vi "Main.vi"(8 "error in":errorcluster) -> (0 "error out":errorcluster)   [LabVIEW 2018, in "Covers-o-meter.lvlib"]
doc: "This module is a free standing module of the car wash.\nIt can be stopped by the 'stop all' user event and has \na QMH architcture. The controller communicates with\nit via its named queue."
uses:
  Covers-o-meter.lvlib
  Private/ctl/Start pause toggle button--boolean.ctl
  Private/ctl/State--enum.ctl
  Private/ctl/Project--cluster.ctl
  Private/ctl/Requirements--cluster.ctl
  <vilib>/National Instruments/Simple DVR Timer API/Timer.lvclass
  Private/ctl/Queue action--enum.ctl
  <vilib>/NI/Timer/Timer Session.lvclass
panel:
  in  "Scan period (min)":dbl[unit]=300.0 format="%#_13g"
  out "Tree 2":string[](tree)
  in  "Reset Button":bool
  out "Cluster":T3
  out "Time left":string
  out "State":T4
  in  "Projects":u16(ring) items=["Car_wash_attempt_2_LE.lvproj", "CLA Covers-o-meter.lvproj"]
  in  "In progress?":T5
  in  "Path to Requirements Tags":path=path "C:/Users/theta/OneDrive/Desktop/CLA/Tools/Sandbox/Data/ATM Requirements Tag.txt"
  out "Coverage over time":waveform(dbl)(graph)
  out "Requirements covered":i32(knob) scale=0.0..103.0
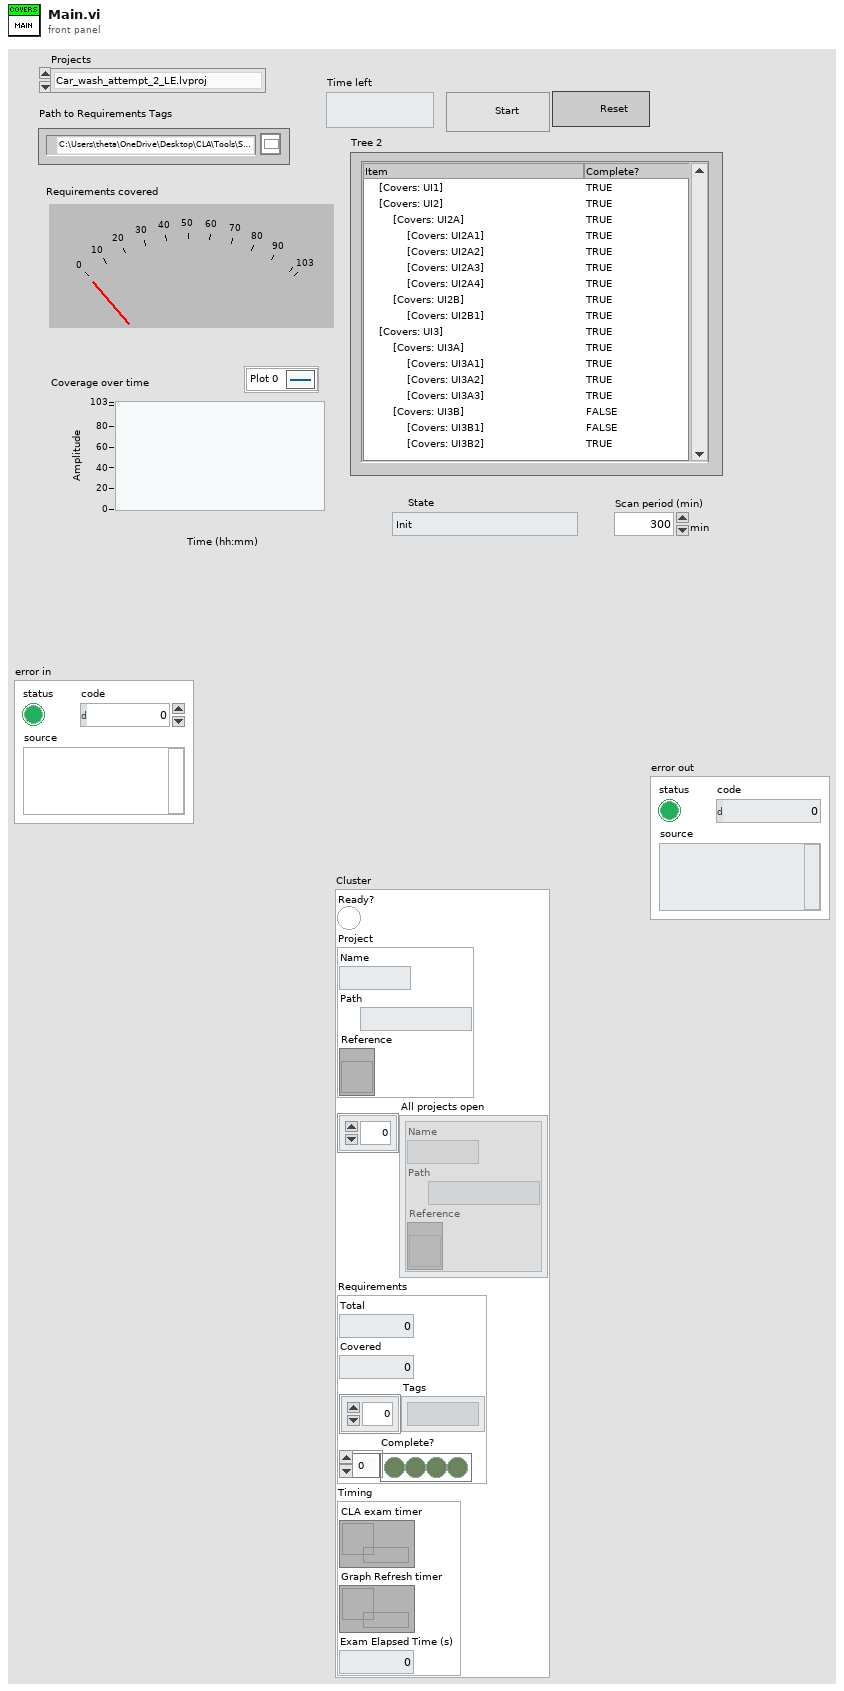
[diagram p1: front panel]
types:
  T1 = typedef "Covers-o-meter.lvlib/Project--cluster.ctl" = cluster{"Name":string, "Path":path, "Reference":refnum<vi>}
  T2 = typedef "Covers-o-meter.lvlib/Requirements--cluster.ctl" = cluster{"Total":i32, "Covered":i32, "Tags":string[], "Complete?":bool[]}
  T3 = cluster{"Ready?":bool, "Project":T1, "All projects open":T1[], "Requirements":T2, "Timing":cluster{"CLA exam timer":refnum<data-value>, "Graph Refresh timer":refnum<data-value>, "Exam Elapsed Time (s)":dbl}}
  T4 = typedef "Covers-o-meter.lvlib/State--enum.ctl" = enum16{"Init", "Init: Read req tags", "Init Data: All Projects", "Init: Which Project?", "Update Requirements tags", "Get all project strings", "Search proj for tags", "Subroutine", "Update Project", "Start Button Pressed", "Start timer", "Error", "Close", "UI - Refresh Timer ", "UI - refresh graph", "UI - Refresh Tree"}
  T5 = typedef "Covers-o-meter.lvlib/Start pause toggle button--boolean.ctl" = bool
  T6 = cluster{"VI Description":bool, "Project Description":bool, "Library Description":bool, "Text within VI":bool, "Class Description":bool}
  T7 = typedef "Covers-o-meter.lvlib/Queue action--enum.ctl" = enum16{"Create", "Get", "Destroy"}
  T8 = typedef "Covers-o-meter.lvlib/Message--enum.ctl" = cluster{"State":T4, "Data":variant}
  T9 = enum8{"Enabled", "Disabled", "Disabled and Grayed Out"}
  T10 = typedef "Start pause toggle button--boolean.ctl" = bool
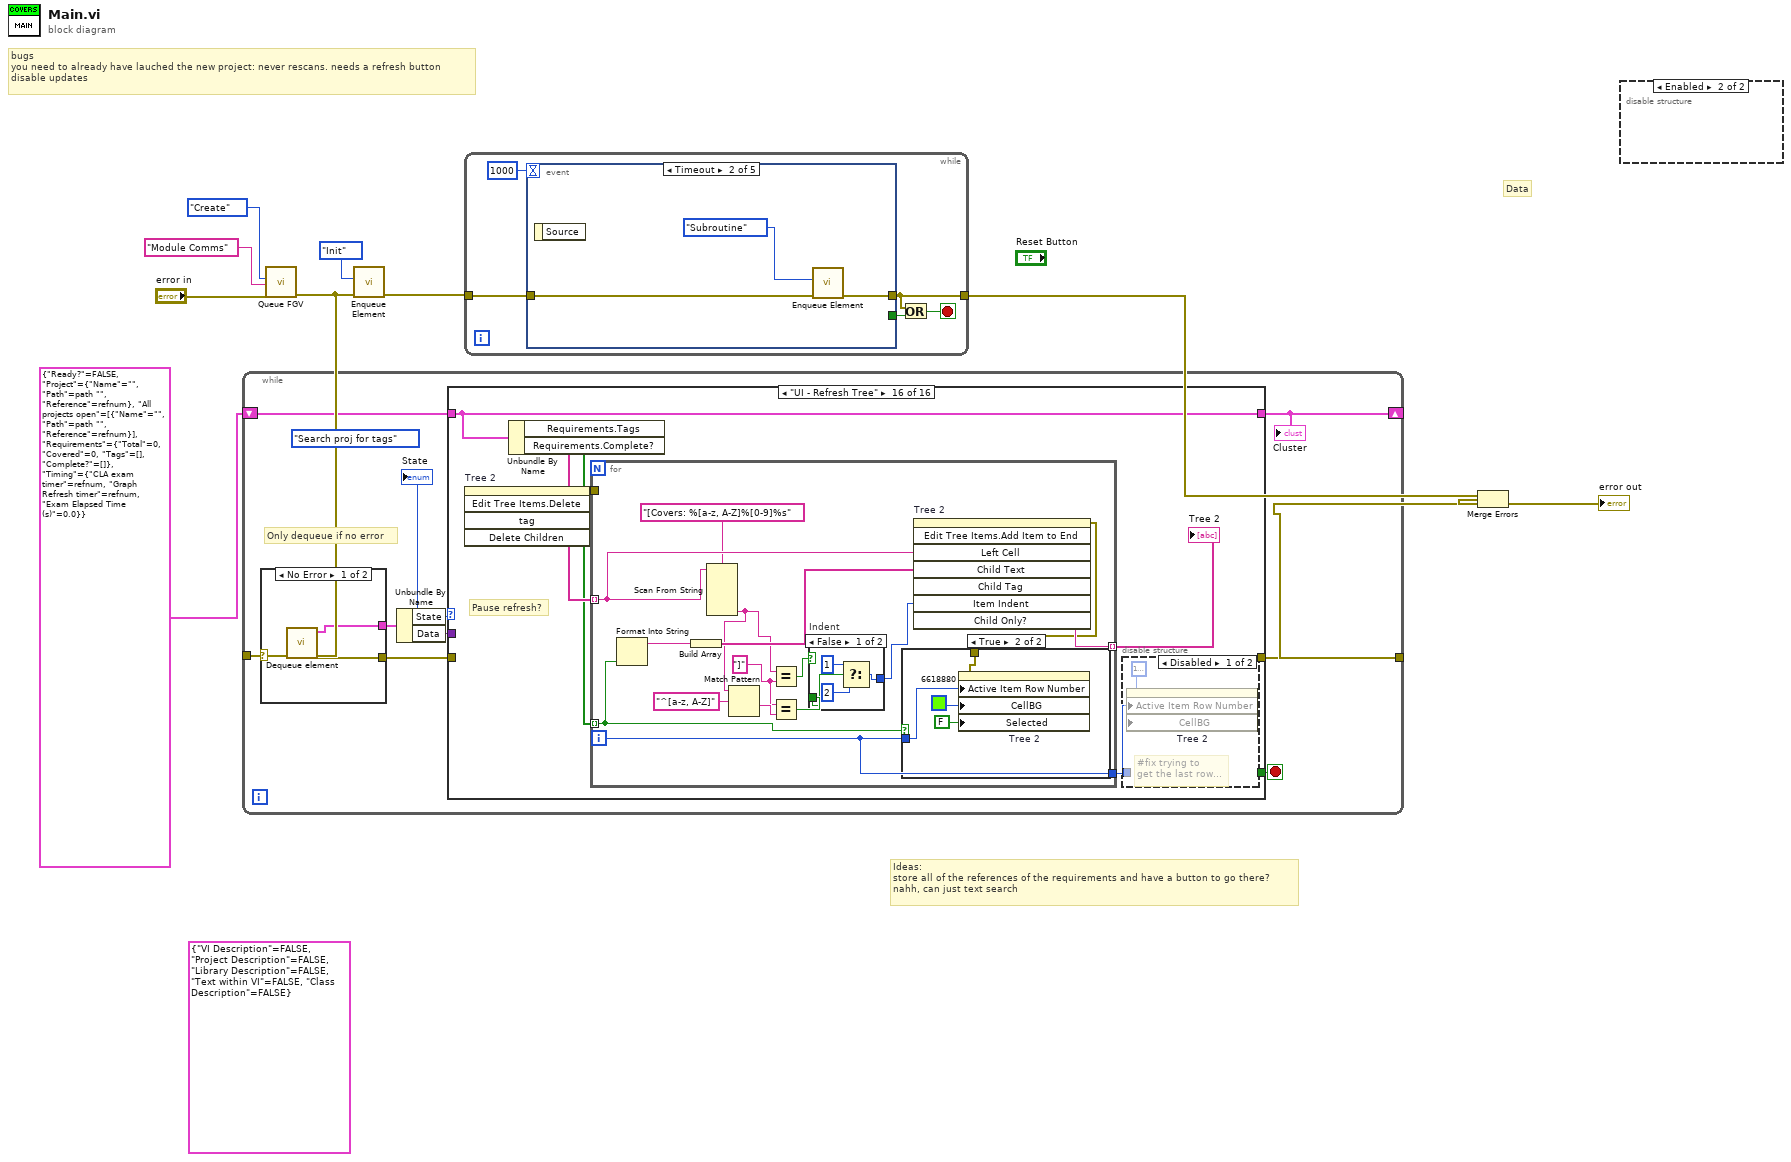
[diagram p0: block diagram]
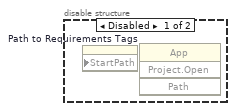
[diagram p2: hidden frame]
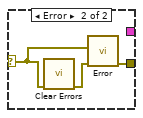
[diagram p3: hidden frame]
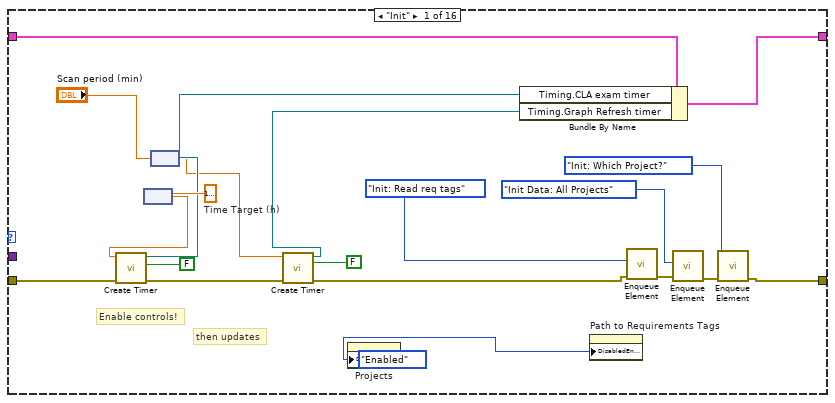
[diagram p4: hidden frame]
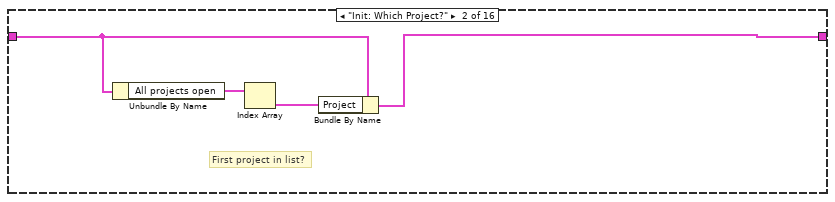
[diagram p5: hidden frame]
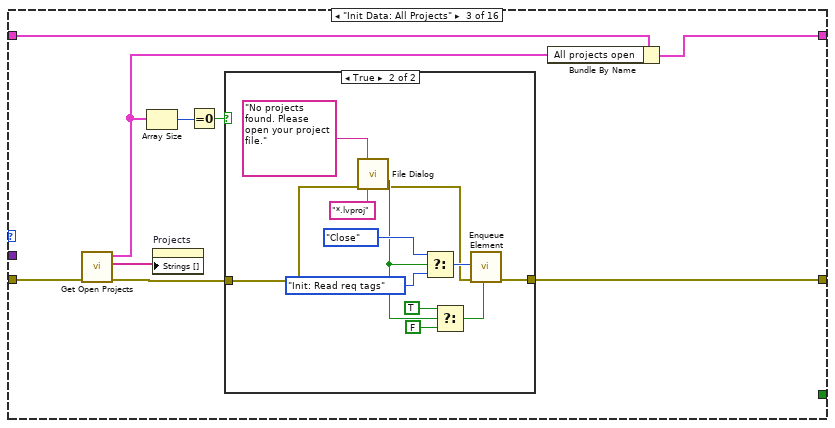
[diagram p6: hidden frame]
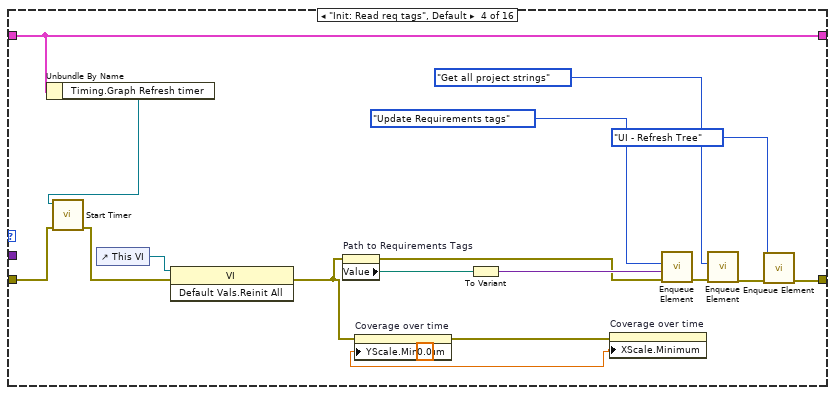
[diagram p8: hidden frame]
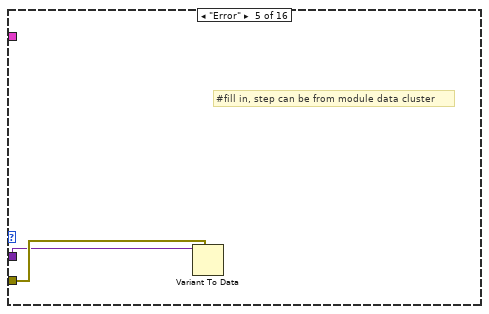
[diagram p9: hidden frame]
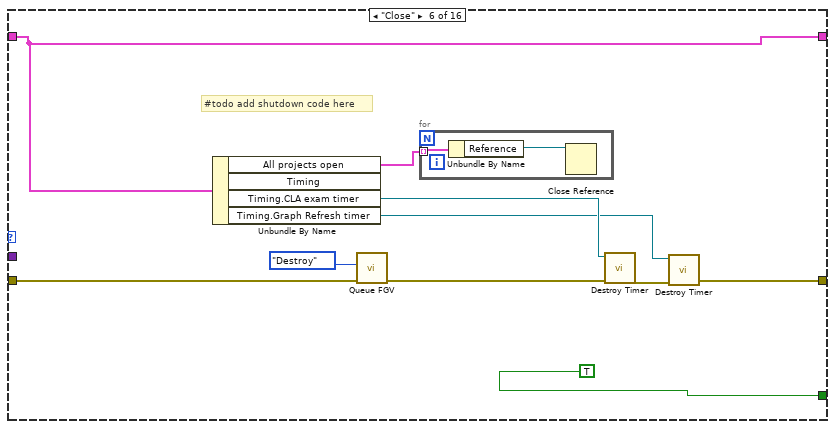
[diagram p10: hidden frame]
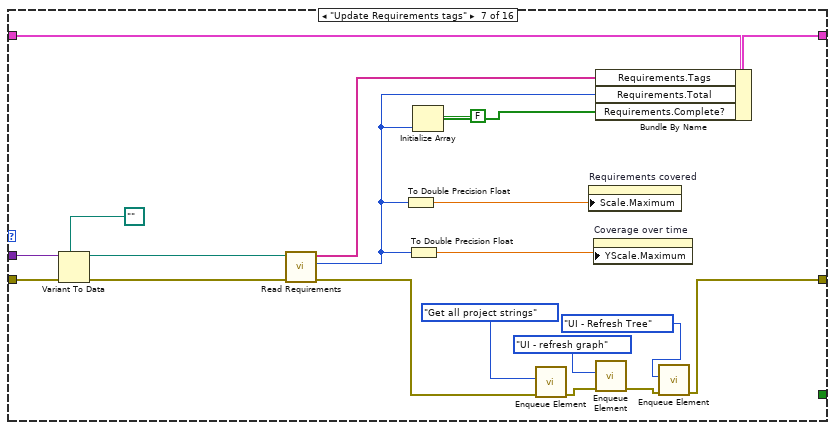
[diagram p11: hidden frame]
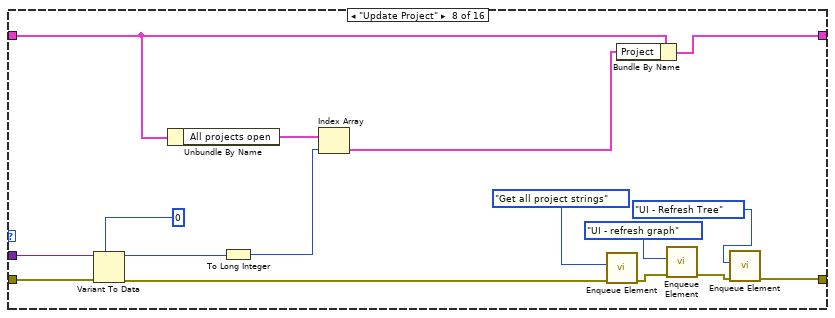
[diagram p12: hidden frame]
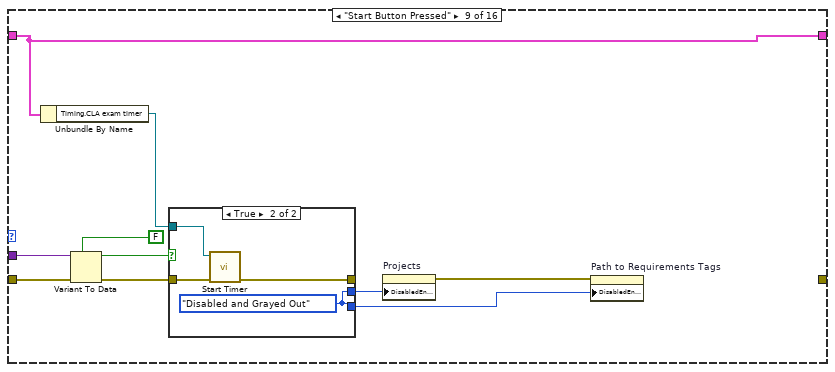
[diagram p13: hidden frame]
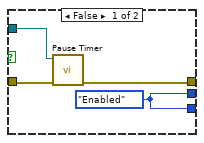
[diagram p14: hidden frame]
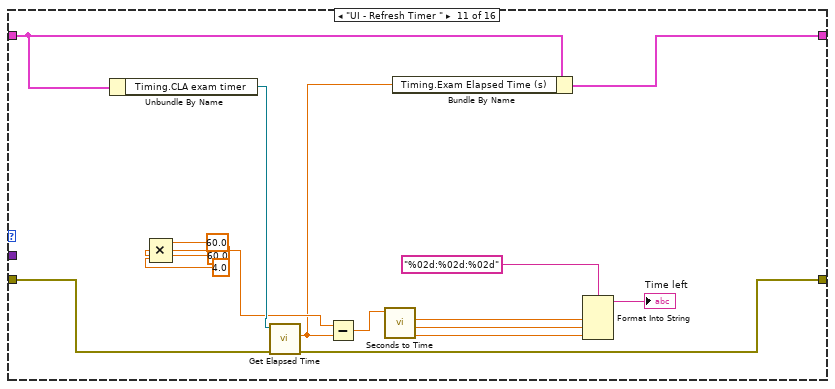
[diagram p16: hidden frame]
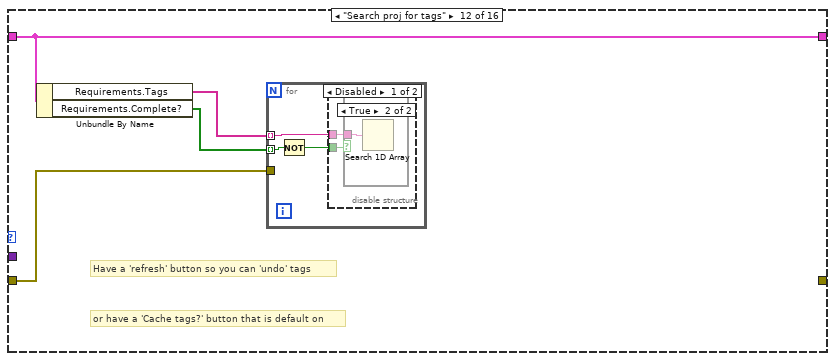
[diagram p17: hidden frame]
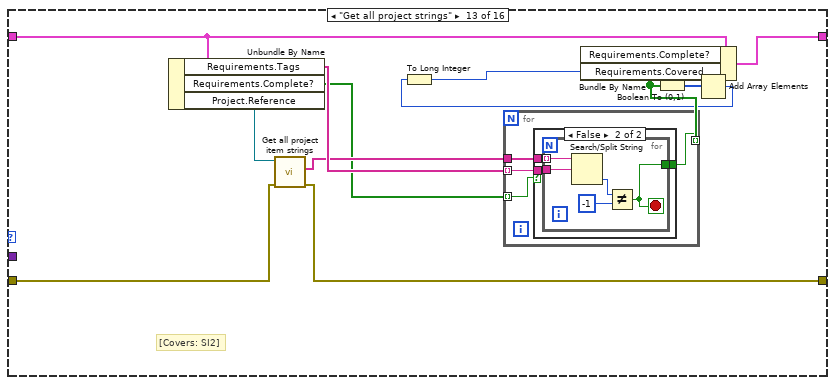
[diagram p20: hidden frame]
diagram:
  (unwired) T6 {"VI Description"=FALSE, "Project Description"=FALSE, "Library Description"=FALSE, "Text within VI"=FALSE, "Class Description"=FALSE}
  # "bugs\nyou need to already have lauched the new project: never rescans. needs a refresh button\ndisable updates"
  # "Ideas:\nstore all of the references of the requirements and have a button to go there?\nnahh, can just text search"
  # "Data"
  n1 = call "Queue FGV.vi"("error in"="error in", "Queue name (unnamed)"="Module Comms", "Queue Action"=Queue_action--enum."Create") -> ("error out"=w7:errorcluster)  [unwired: 7 in, 1 out]
  n2 = while {
    tunnel: [w16] -> w1
    shift-right: [w11] -> _
    shift-left: T3 {"Ready?"=FALSE, "Project"={"Name"="", "Path"=path "", "Reference"=refnum}, "All projects open"=[{"Name"="", "Path"=path "", "Reference"=refnum}], "Requirements"={"Total"=0, "Covered"=0, "Tags"=[], "Complete?"=[]}, "Timing"={"CLA exam timer"=refnum, "Graph Refresh timer"=refnum, "Exam Elapsed Time (s)"=0.0}} -> [w12]
    tunnel: w7 -> [w13]
    stop <- w15 stop-if-true
    (unwired) State--enum."Search proj for tags" ("State")
    # "Only dequeue if no error"
    n3 = case shown="No Error" w13 {
      selector: w13 -> [w21 w23]
      tunnel: [w22 w25] -> w17
      tunnel: [w20 _] -> w19
      frame No Error {
        n4 = call "Dequeue element.vi"("error in (no error)"=w21) -> ("error out"=w22:errorcluster, "Message"=w20:T8)  [unwired: 9 in]
      }
      frame Error {
        n5 = call <vilib>:"Clear Errors.vi"("error in (no error)"=w23) -> ("error out"=w24:errorcluster)  [unwired: 5 in, 1 out]
        n6 = call "Error.vi"("error in (no error)"=w24, "error to pass"=w23) -> ("error out"=w25:errorcluster)  [unwired: 9 in]
      }
    }
    n7 = Unbundle By Name(w19) -> ("State"=w18:T4, "Data"=w14:variant)
    "State" <- w18
    n8 = case shown="\"UI - Refresh Tree\"" w18 {
      tunnel: w17 -> [w40 _ w56 w78 w90 w99 w120 w138 w147 _ w162 w176 w184 w212 w238 _]
      tunnel: [w41 _ w51 w74 _ w91 w103 w124 _ _ w161 _ w195 w213 w237 _] -> w16
      tunnel: [_ _ _ _ _ TRUE _ _ _ _ _ _ _ _ _ _] -> w15
      tunnel: w14 -> [_ _ _ _ w89 _ w121 w137 w146 _ _ _ _ _ _ _]
      tunnel: [w35 w46 w50 w81 _ w95 w117 w132 w142 w157 w158 w174 w190 w217 w235 w242] -> w11
      tunnel: w12 -> [w34 w49 w57 w81 _ w95 w116 w134 w142 w157 w159 w174 w194 w217 w235 w242]
      frame "Init" {
        w26 = T9."Enabled" ("Disabled")
        w39 = dbl[unit] 14400.0  # Time Target (h)
        # "Enable controls!"
        # "then updates"
        n9 = node(w39) -> (w38:dbl)
        n10 = call <vilib>:"Create Timer.vi"("Error In"=w40, "Auto-reset on Time Elapsed"=FALSE, "Time Goal (s)"=w38) -> ("Error Out"=w29:errorcluster, "Timer Reference"=w36:refnum<data-value>)  [unwired: 7 in]
        n11 = node("Scan period (min)") -> (w30:dbl)
        n12 = call <vilib>:"Create Timer.vi"("Error In"=w29, "Auto-reset on Time Elapsed"=FALSE, "Time Goal (s)"=w30) -> ("Error Out"=w32:errorcluster, "Timer Reference"=w27:refnum<data-value>)  [unwired: 7 in]
        n13 = property on="Projects" class="Ring (strict)"("DisabledEnum"=w26) -> ()  [unwired: 2 in, 2 out]
        n14 = Bundle By Name(cluster=w34, "Timing.CLA exam timer"=w36, "Timing.Graph Refresh timer"=w27) -> (w35:T3)
        n15 = property on="Path to Requirements Tags" class="Path"("DisabledEnum"=w26) -> ()  [unwired: 2 in, 2 out]
        n16 = call "Enqueue Element.vi"("error in"=w32, "State"=State--enum."Init: Read req tags") -> ("error out"=w33:errorcluster)  [unwired: 9 in]
        n17 = call "Enqueue Element.vi"("error in"=w33, "State"=State--enum."Init Data: All Projects") -> ("error out"=w43:errorcluster)  [unwired: 9 in]
        n18 = call "Enqueue Element.vi"("error in"=w43, "State"=State--enum."Init: Which Project?") -> ("error out"=w41:errorcluster)  [unwired: 9 in]
      }
      frame "Init: Which Project?" {
        # "First project in list?"
        n19 = Unbundle By Name(w49) -> ("All projects open"=w48:T1[])
        n20 = Index Array(array=w48) -> (element=w47:T1)  [unwired: 1 in]
        n21 = Bundle By Name(cluster=w49, "Project"=w47) -> (w46:T3)
      }
      frame "Init Data: All Projects" {
        n22 = call "Get Open Projects.vi"("error in (no error)"=w56) -> ("error out"=w52:errorcluster, "Project Names"=w58:string[], "Project Data"=w55:T1[])  [unwired: 8 in]
        n23 = Array Size(array=w55) -> (size(s)=w54:i32)
        n24 = property on="Projects" class="Ring (strict)"("Strings []"=w58) -> ()  [unwired: 2 in, 2 out]
        n25 = Equal To 0?(x=w54) -> (x = 0?=w53:bool)
        n26 = case shown="True" w53 {
          tunnel: w52 -> [w59 w62]
          tunnel: [w59 w60] -> w51
          frame False {
            # "It's okay, there's\na project open"
          }
          frame True {
            n27 = call "File Dialog"("prompt"="No projects found. Please open your project file.", "error in"=w62, "pattern (all files)"="*.lvproj") -> ("cancelled"=w66:bool, "error out"=w61:errorcluster)  [unwired: 9 in, 2 out]
            n28 = Select(t=State--enum."Close" ("State"), s=w66, f=State--enum."Init: Read req tags" ("State")) -> (s? t:f=w67:T4)
            n29 = Select(t=TRUE, s=w66, f=FALSE) -> (s? t:f=w64:bool)
            n30 = call "Enqueue Element.vi"("Priority? (F)"=w64, "error in"=w61, "State"=w67) -> ("error out"=w60:errorcluster)  [unwired: 8 in]
          }
        }
        n31 = Bundle By Name(cluster=w57, "All projects open"=w55) -> (w50:T3)
      }
      frame "Init: Read req tags", Default {
        w76 = 0.0 ("Y Scale.Range:Minimum")
        n32 = Unbundle By Name(w81) -> ("Timing.Graph Refresh timer"=w80:refnum<data-value>)
        n33 = call <vilib>:"Start Timer.vi"("Error In"=w78, "Timer Reference"=w80) -> ("Error Out"=w79:errorcluster)  [unwired: 8 in, 1 out]
        n34 = control-ref of="This VI"() -> (w88:refnum<vi>)
        n35 = invoke class="VI" method="Default Vals.Reinit All"(reference=w88, error in=w79) -> (error out=w77:errorcluster)  [unwired: 1 in, 2 out]
        n36 = property on="Path to Requirements Tags" class="Path"(error in=w77) -> (error out=w84:errorcluster, "Value"=w85:path)  [unwired: 1 in, 1 out]
        n37 = property on="Coverage over time" class="WFChart (strict)"(error in=w77, "YScale.Minimum"=w76) -> (error out=w75:errorcluster)  [unwired: 1 in, 1 out]
        n38 = To Variant(anything=w85) -> (Variant=w87:variant)
        n39 = property on="Coverage over time" class="WFChart (strict)"(error in=w75, "XScale.Minimum"=w76) -> ()  [unwired: 1 in, 2 out]
        n40 = call "Enqueue Element.vi"("error in"=w84, "Data"=w87, "State"=State--enum."Update Requirements tags") -> ("error out"=w83:errorcluster)  [unwired: 8 in]
        n41 = call "Enqueue Element.vi"("error in"=w83, "State"=State--enum."Get all project strings") -> ("error out"=w73:errorcluster)  [unwired: 9 in]
        n42 = call "Enqueue Element.vi"("error in"=w73, "State"=State--enum."UI - Refresh Tree") -> ("error out"=w74:errorcluster)  [unwired: 9 in]
      }
      frame "Error" {
        # "#fill in, step can be from module data cluster"
        n43 = Variant To Data(type=w90, Variant=w89) -> ()  [unwired: 1 in, 2 out]
      }
      frame "Close" {
        # "#todo add shutdown code here"
        n44 = Unbundle By Name(w95) -> ("All projects open"=w92:T1[], "Timing.CLA exam timer"=w97:refnum<data-value>, "Timing.Graph Refresh timer"=w93:refnum<data-value>)  [unwired: 1 out]
        n45 = call "Queue FGV.vi"("error in"=w99, "Queue Action"=Queue_action--enum."Destroy") -> ("error out"=w96:errorcluster)  [unwired: 8 in, 1 out]
        n46 = for {
          tunnel: w92 -> [w102] mode=indexing
          n47 = Unbundle By Name(w102) -> ("Reference"=w101:refnum<vi>)
          n48 = Close Reference(reference=w101) -> ()  [unwired: 1 in, 1 out]
        }
        n49 = call <vilib>:"Destroy Timer.vi"("Error In"=w96, "Timer In"=w97) -> ("Error Out"=w94:errorcluster)  [unwired: 8 in, 1 out]
        n50 = call <vilib>:"Destroy Timer.vi"("Error In"=w94, "Timer In"=w93) -> ("Error Out"=w91:errorcluster)  [unwired: 8 in, 1 out]
      }
      frame "Update Requirements tags" {
        n51 = Variant To Data(error in=w120, type=path "", Variant=w121) -> (data=w119:path, error out=w118:errorcluster)
        n52 = call "Read Requirements.vi"("error in (no error)"=w118, "Requirements file"=w119) -> ("error out"=w104:errorcluster, "# Requirements"=w110:i32, "Requirements"=w115:string[])  [unwired: 7 in]
        n53 = To Double Precision Float(number=w110) -> (double precision float=w112:dbl)
        n54 = To Double Precision Float(number=w110) -> (double precision float=w111:dbl)
        n55 = Initialize Array(FALSE, w110) -> (w114:bool[])
        n56 = call "Enqueue Element.vi"("error in"=w104, "State"=State--enum."Get all project strings") -> ("error out"=w106:errorcluster)  [unwired: 9 in]
        n57 = property on="Requirements covered" class="Knob (strict)"("Scale.Maximum"=w112) -> ()  [unwired: 2 in, 2 out]
        n58 = property on="Coverage over time" class="WFChart (strict)"("YScale.Maximum"=w111) -> ()  [unwired: 2 in, 2 out]
        n59 = Bundle By Name(cluster=w116, "Requirements.Tags"=w115, "Requirements.Total"=w110, "Requirements.Complete?"=w114) -> (w117:T3)
        n60 = call "Enqueue Element.vi"("error in"=w106, "State"=State--enum."UI - refresh graph") -> ("error out"=w108:errorcluster)  [unwired: 9 in]
        n61 = call "Enqueue Element.vi"("error in"=w108, "State"=State--enum."UI - Refresh Tree") -> ("error out"=w103:errorcluster)  [unwired: 9 in]
      }
      frame "Update Project" {
        n62 = Variant To Data(error in=w138, type=u16 0 ("NewVal"), Variant=w137) -> (data=w130:u16, error out=w125:errorcluster)
        n63 = Unbundle By Name(w134) -> ("All projects open"=w135:T1[])
        n64 = To Long Integer(number=w130) -> (32bit integer=w131:i32)
        n65 = Index Array(array=w135, index=w131) -> (element=w133:T1)
        n66 = call "Enqueue Element.vi"("error in"=w125, "State"=State--enum."Get all project strings") -> ("error out"=w126:errorcluster)  [unwired: 9 in]
        n67 = Bundle By Name(cluster=w134, "Project"=w133) -> (w132:T3)
        n68 = call "Enqueue Element.vi"("error in"=w126, "State"=State--enum."UI - refresh graph") -> ("error out"=w128:errorcluster)  [unwired: 9 in]
        n69 = call "Enqueue Element.vi"("error in"=w128, "State"=State--enum."UI - Refresh Tree") -> ("error out"=w124:errorcluster)  [unwired: 9 in]
      }
      frame "Start Button Pressed" {
        n70 = Unbundle By Name(w142) -> ("Timing.CLA exam timer"=w143:refnum<data-value>)
        n71 = Variant To Data(error in=w147, type=FALSE, Variant=w146) -> (data=w144:bool, error out=w148:errorcluster)
        n72 = case shown="True" w144 {
          tunnel: [w152 w156] -> _
          tunnel: w148 -> [w151 w155]
          tunnel: w143 -> [w150 w154]
          tunnel: [w149 w153] -> w140
          tunnel: [w149 w153] -> w139
          frame False {
            w149 = T9."Enabled" ("Disabled")
            n73 = call <vilib>:"Pause Timer.vi"("Error In"=w151, "Timer Reference"=w150) -> ("Error Out"=w152:errorcluster)  [unwired: 8 in, 1 out]
          }
          frame True {
            w153 = T9."Disabled and Grayed Out" ("Disabled")
            n74 = call <vilib>:"Start Timer.vi"("Error In"=w155, "Timer Reference"=w154) -> ("Error Out"=w156:errorcluster)  [unwired: 8 in, 1 out]
          }
        }
        n75 = property on="Projects" class="Ring (strict)"("DisabledEnum"=w140) -> (error out=w141:errorcluster)  [unwired: 2 in, 1 out]
        n76 = property on="Path to Requirements Tags" class="Path"(error in=w141, "DisabledEnum"=w139) -> ()  [unwired: 1 in, 2 out]
      }
      frame "Start timer" {
      }
      frame "UI - Refresh Timer " {
        n77 = Unbundle By Name(w159) -> ("Timing.CLA exam timer"=w172:refnum<data-value>)
        n78 = Compound Arithmetic op=MULTIPLY(60.0 ("value"), 60.0 ("value"), 4.0 ("value")) -> (w163:dbl)
        n79 = call <vilib>:"Get Elapsed Time.vi"("Error In"=w162, "Timer Reference"=w172) -> ("Error Out"=w161:errorcluster, "Elapsed Time (s)"=w160:dbl)  [unwired: 6 in, 2 out]
        n80 = Subtract(x=w163, y=w160) -> (x-y=w167:dbl)
        n81 = call <vilib>:"Seconds to Time.vi"("Time Goal (s)"=w167) -> ("Seconds"=w169:dbl, "Minutes"=w170:dbl, "Hours"=w168:dbl)  [unwired: 7 in, 1 out]
        n82 = Bundle By Name(cluster=w159, "Timing.Exam Elapsed Time (s)"=w160) -> (w158:T3)
        n83 = Format Into String(format string="%02d:%02d:%02d", w168, w170, w169) -> (resulting string=→"Time left":string)  [unwired: 2 in, 1 out]
      }
      frame "Search proj for tags" {
        # "or have a 'Cache tags?' button that is default on"
        # "Have a 'refresh' button so you can 'undo' tags"
        n84 = Unbundle By Name(w174) -> ("Requirements.Tags"=w177:string[], "Requirements.Complete?"=w175:bool[])
        n85 = for {
          tunnel: w177 -> [w178] mode=indexing
          tunnel: w176 -> [_]
          tunnel: w175 -> [w180] mode=indexing
          n86 = Not(x=w180) -> (.not. x?=w179:bool)
          n87 = disable-structure shown="Disabled" {
            disable-tunnel: w179 -> [w182 _]
            disable-tunnel: w178 -> [w181 _]
            frame Disabled {
              n88 = case shown="True" w182 {
                tunnel: w181 -> [_ w183]
                frame False {
                }
                frame True {
                  n89 = Search 1D Array(element=w183) -> ()  [unwired: 2 in, 1 out]
                }
              }
            }
            frame Enabled {
            }
          }
        }
      }
      frame "Get all project strings" {
        # "[Covers: SI2]"
        n90 = Unbundle By Name(w194) -> ("Requirements.Tags"=w193:string[], "Requirements.Complete?"=w191:bool[], "Project.Reference"=w185:refnum<vi>)
        n91 = call "Get all project item strings.vi"("error in (no error)"=w184, "Project.Reference"=w185) -> ("error out"=w195:errorcluster, "All Strings"=w192:string[])  [unwired: 8 in]
        n92 = for {
          tunnel: w193 -> [w199] mode=indexing
          tunnel: w192 -> [w198]
          tunnel: [w197] -> w188 mode=indexing
          tunnel: w191 -> [w196] mode=indexing
          n93 = case shown="False" w196 {
            selector: w196 -> [w200 _]
            tunnel: w199 -> [_ w203]
            tunnel: w198 -> [_ w202]
            tunnel: [w200 w201] -> w197
            frame True {
              # "No need to search"
            }
            frame False {
              n94 = for {
                tunnel: w203 -> [w208]
                tunnel: w202 -> [w207] mode=indexing
                tunnel: [w204] -> w201
                stop <- w204 stop-if-true
                n95 = Search/Split String(string=w207, search string/char (-)=w208) -> (offset of match=w206:i32)  [unwired: 1 in, 2 out]
                n96 = Not Equal?(x=w206, y=-1) -> (x != y?=w204:bool)
              }
            }
          }
        }
        n97 = Boolean To (0,1)(Boolean=w188) -> (0, 1=w189:i16[])
        n98 = Add Array Elements(numeric array=w189) -> (sum=w186:i16)
        n99 = To Long Integer(number=w186) -> (32bit integer=w187:i32)
        n100 = Bundle By Name(cluster=w194, "Requirements.Complete?"=w188, "Requirements.Covered"=w187) -> (w190:T3)
      }
      frame "Subroutine" {
        # "AND play?"
        n101 = Unbundle By Name(w217) -> ("Timing.Graph Refresh timer"=w215:refnum<data-value>)
        n102 = call "Enqueue Element.vi"("error in"=w212, "State"=State--enum."UI - Refresh Timer ") -> ("error out"=w216:errorcluster)  [unwired: 9 in]
        n103 = call <vilib>:"Get Elapsed Time.vi"("Error In"=w216, "Timer Reference"=w215) -> ("Error Out"=w214:errorcluster, "Time Has Elapsed"=w210:bool)  [unwired: 6 in, 2 out]
        n104 = property on="In progress?" class="Bool (strict)"() -> ("Value"=w211:T10)  [unwired: 2 in, 2 out]
        n105 = And(x=w211, y=w210) -> (x .and. y?=w209:T10)
        n106 = case shown="True" w209 {
          tunnel: w214 -> [w219 w221]
          tunnel: [w219 w225] -> w213
          frame False {
          }
          frame True {
            n107 = call "Enqueue Element.vi"("error in"=w221, "State"=State--enum."Get all project strings") -> ("error out"=w220:errorcluster)  [unwired: 9 in]
            n108 = call "Enqueue Element.vi"("error in"=w220, "State"=State--enum."UI - refresh graph") -> ("error out"=w224:errorcluster)  [unwired: 9 in]
            n109 = call "Enqueue Element.vi"("error in"=w224, "State"=State--enum."UI - Refresh Tree") -> ("error out"=w225:errorcluster)  [unwired: 9 in]
          }
        }
      }
      frame "UI - refresh graph" {
        n110 = Unbundle By Name(w235) -> ("Requirements.Covered"=w234:i32, "Timing.Graph Refresh timer"=w236:refnum<data-value>, "Timing.Exam Elapsed Time (s)"=w228:dbl)
        "Requirements covered" <- w234
        n111 = call <vilib>:"Reset Timer.vi"("Error In"=w238, "Timer Reference"=w236) -> ("Error Out"=w237:errorcluster)  [unwired: 8 in, 1 out]
        n112 = To Double Precision Float(number=w234) -> (double precision float=w227:dbl)
        n113 = Divide(x=w228, y=60.0) -> (x/y=w232:dbl)
        n114 = Build Array(w232, w227) -> ()  [unwired: 1 out]
        n115 = To Time Stamp(1:w228) -> (0:w230:timestamp)
        n116 = Seconds To Date/Time() -> ()  [unwired: 2 in, 1 out]
        n117 = Build Array(w227) -> (w229:dbl[])
        n118 = Bundle By Name("Y"=w229, "t0"=w230) -> (→"Coverage over time":waveform(dbl))  [unwired: 1 in]
      }
      frame "UI - Refresh Tree" {
        # "Pause refresh?"
        n119 = invoke on="Tree 2" class="Tree (strict)" method="Edit Tree Items.Delete"() -> (error out=w241:errorcluster)  [unwired: 5 in, 4 out]
        n120 = Unbundle By Name(w242) -> ("Requirements.Tags"=w244:string[], "Requirements.Complete?"=w243:bool[])
        n121 = for {
          tunnel: w244 -> [w261] mode=indexing
          tunnel: [w259] -> w240 mode=indexing
          tunnel: w243 -> [w249] mode=indexing
          tunnel: w241 -> [_]
          tunnel: [w247] -> w239
          i -> [w247]
          w250 = "]" ("y")
          n122 = Format Into String(w249) -> (resulting string=w254:string)  [unwired: 3 in, 1 out]
          n123 = Build Array(w254) -> (w258:string[])
          n124 = Scan From String(format string="[Covers: %[a-z, A-Z]%[0-9]%s", input string=w261) -> (output 3=w257:string)  [unwired: 7 in, 3 out]
          n125 = Match Pattern(string=w257, regular expression="^[a-z, A-Z]") -> (after substring=w253:string)  [unwired: 1 in, 3 out]
          n126 = Equal?(x=w257, y=w250) -> (x = y?=w252:bool)
          n127 = Equal?(x=w250, y=w253) -> (x = y?=w251:bool)
          n128 = case "Indent" shown="False" w252 {
            tunnel: [w272 0 ("Numeric")] -> w260
            tunnel: w251 -> [w271 _]
            frame False {
              n129 = Select(t=1 ("Numeric"), s=w271, f=2 ("Numeric")) -> (s? t:f=w272:i32)
            }
            frame True {
            }
          }
          n130 = invoke on="Tree 2" class="Tree (strict)" method="Edit Tree Items.Add Item to End"("Left Cell"=w261, "Child Text"=w258, "Item Indent"=w260) -> (error out=w248:errorcluster, "Edit Tree Items:Add Item to End"=w259:string)  [unwired: 5 in, 6 out]
          n131 = case shown="True" w249 {
            tunnel: w248 -> [w266 w268]
            tunnel: w247 -> [w265 w270]
            frame False {
              w263 = u32 16777225
              n132 = property on="Tree 2" class="Tree (strict)"(error in=w266, "Active Item Row Number"=w265, "CellBG"=w263, "SelectEntireRows"=FALSE ("Select Entire Rows"), "SelColor"=w263, "Selected"=FALSE) -> ()  [unwired: 1 in, 2 out]
            }
            frame True {
              n133 = property on="Tree 2" class="Tree (strict)"(error in=w268, "Active Item Row Number"=w270, "CellBG"=u32 6618880, "Selected"=FALSE) -> ()  [unwired: 1 in, 2 out]
            }
          }
        }
        "Tree 2" <- w240
        n134 = disable-structure shown="Disabled" {
          disable-tunnel: w239 -> [w246 _]
          frame Disabled {
            # "#fix trying to \nget the last row..."
            n135 = property on="Tree 2" class="Tree (strict)"("Active Item Row Number"=w246, "CellBG"=u32 16777225) -> ()  [unwired: 2 in, 2 out]
          }
          frame Enabled {
          }
        }
      }
    }
    "Cluster" <- w11
  }
  n136 = call "Enqueue Element.vi"("error in"=w7, "State"=State--enum."Init") -> ("error out"=w2:errorcluster)  [unwired: 9 in]
  n137 = while {
    tunnel: w2 -> [w278]
    tunnel: [w277] -> w4
    stop <- w280 stop-if-true
    n138 = event shown="[1] Timeout" {
      selector: _ -> [_ _ _ _ _]
      dyn-events: _ -> [_ _ _ _ _]
      timeout: 1000 -> [_ _ _ _ _]
      tunnel: [TRUE _ _ _ _] -> w279
      tunnel: w278 -> [_ w282 w288 w296 w299]
      tunnel: [_ w283 w287 w292 w298] -> w277
      event Panel Close {
        n139 = event-data() -> ()  [unwired: 1 in, 4 out]
      }
      event Timeout {
        n140 = event-data() -> ()  [unwired: 1 in, 1 out]
        n141 = call "Enqueue Element.vi"("error in"=w282, "State"=State--enum."Subroutine") -> ("error out"=w283:errorcluster)  [unwired: 9 in]
      }
      event "Projects": Value Change {
        n142 = event-data() -> ("NewVal"=w290:u16)  [unwired: 1 in]
        n143 = To Variant(anything=w290) -> (Variant=w289:variant)
        n144 = call "Enqueue Element.vi"("error in"=w288, "Data"=w289, "State"=State--enum."Update Project") -> ("error out"=w286:errorcluster)  [unwired: 8 in]
        n145 = call "Enqueue Element.vi"("error in"=w286, "State"=State--enum."Get all project strings") -> ("error out"=w287:errorcluster)  [unwired: 9 in]
      }
      event "Path to Requirements Tags": Value Change {
        n146 = event-data() -> ("NewVal"=w294:path)  [unwired: 1 in]
        n147 = To Variant(anything=w294) -> (Variant=w295:variant)
        n148 = call "Enqueue Element.vi"("error in"=w296, "Data"=w295, "State"=State--enum."Update Requirements tags") -> ("error out"=w292:errorcluster)  [unwired: 8 in]
      }
      event Value Change {
        n149 = event-data() -> ("NewVal"=w297:T5)  [unwired: 1 in]
        n150 = To Variant(anything=w297) -> (Variant=w301:variant)
        n151 = call "Enqueue Element.vi"("error in"=w299, "Data"=w301, "State"=State--enum."Start Button Pressed") -> ("error out"=w298:errorcluster)  [unwired: 8 in]
      }
    }
    n152 = Or(x=w277, y=w279) -> (x .or. y?=w280:bool)
  }
  n153 = Merge Errors(w4, w1) -> (→"error out":errorcluster)
  n154 = disable-structure shown="Enabled" {
    frame Disabled {
      n155 = property on="Path to Requirements Tags" class="Path" props=["StartPath"]() -> ()  [unwired: 3 in, 2 out]
      n156 = invoke class="App" method="Project.Open"() -> ()  [unwired: 4 in, 4 out]
    }
    frame Enabled {
    }
  }
